vi "MakeChassis.vi"(8 "error in (no error)":errorcluster, 11 "ClassicType in":refnum<class "ClassicType.lvclass">) -> (0 "error out":errorcluster, 3 "ClassicType out":refnum<class "ClassicType.lvclass">)   [LabVIEW 2021, in "ClassicType.lvclass"]
uses:
  ClassicType.lvclass
  C:/Users/chrismadlax/Documents/LabVIEW Data/Project/OOP/GeneralCar/GeneralCar.lvclass
  GeneralCar/GeneralCar.lvclass/GeneralCar.ctl
  GeneralCar/GeneralCar.lvclass
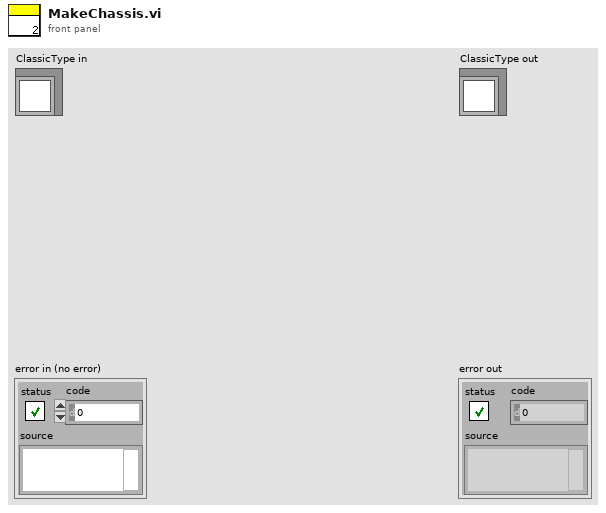
[diagram p1: front panel]
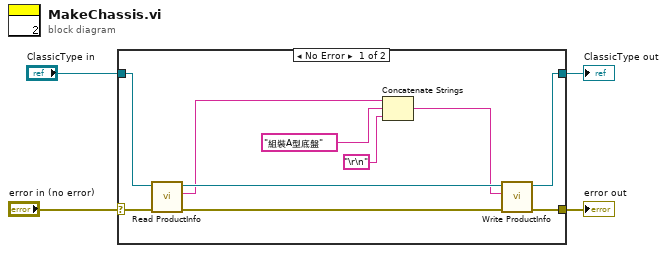
[diagram p0: block diagram]
diagram:
  n1 = case shown="No Error" "error in (no error)" {
    selector: "error in (no error)" -> [w14 w16]
    tunnel: [w11 w16] -> w4
    tunnel: [w9 w15] -> w3
    tunnel: "ClassicType in" -> [w12 w15]
    frame No Error {
      n2 = call "Read ProductInfo.vi"("error in (no error)"=w14, "GeneralCar in"=w12) -> ("error out"=w13:errorcluster, "ProductInfo"=w6:string, "GeneralCar out"=w10:refnum<class "ClassicType.lvclass">)  [unwired: 7 in]
      n3 = Concatenate Strings(w6, "組裝A型底盤" ("string"), "\r\n") -> (w5:string)
      n4 = call "Write ProductInfo.vi"("error in (no error)"=w13, "ProductInfo"=w5, "GeneralCar in"=w10) -> ("error out"=w11:errorcluster, "GeneralCar out"=w9:refnum<class "ClassicType.lvclass">)  [unwired: 7 in]
    }
    frame Error {
    }
  }
  "error out" <- w4
  "ClassicType out" <- w3
